vi "OpenErrorlogFileError.vi"(8 "error in (no error)":errorcluster, 10 "error":errorcluster, 11 "TCP_Client in":refnum<class "TCP_Client.lvclass">) -> (0 "error out":errorcluster, 3 "TCP_Client out":refnum<class "TCP_Client.lvclass">)   [LabVIEW 2023, in "TCP_Client.lvlib" / "TCP_Client.lvclass"]
uses:
  TCP_Client.lvclass
  TCP_Client.lvclass/TCP_Client.ctl
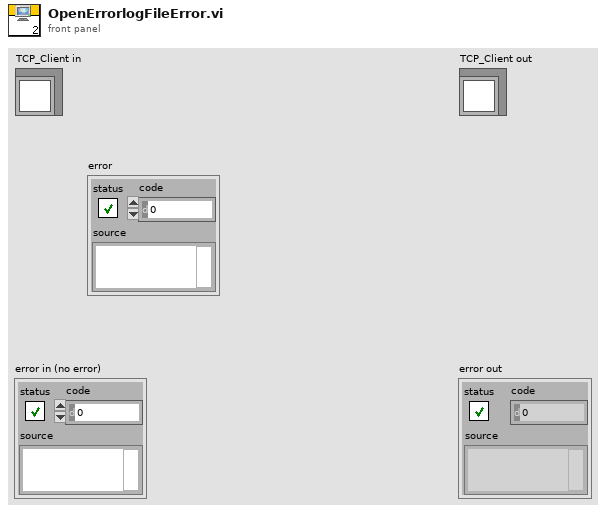
[diagram p1: front panel]
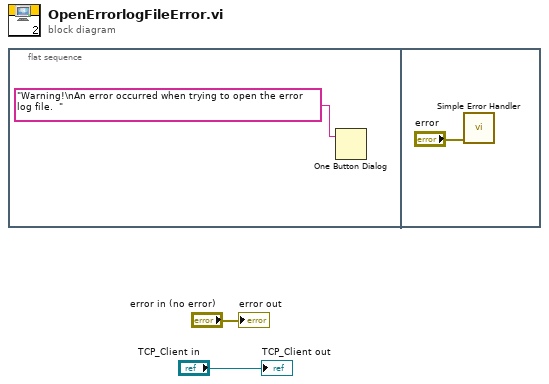
[diagram p0: block diagram]
diagram:
  n1 = flat-sequence {
    frame #0 {
      n2 = One Button Dialog(message="Warning!\nAn error occurred when trying to open the error log file.  ") -> ()  [unwired: 1 in, 1 out]
    }
    frame #1 {
      n3 = call <vilib>:"Simple Error Handler.vi"("error in (no error)"="error") -> ()  [unwired: 4 in, 5 out]
    }
  }
  "error out" <- "error in (no error)"
  "TCP_Client out" <- "TCP_Client in"
